vi "rqcAlice Pulse Detector And DAC Clock (FPGA).vi"(0 "delay line signal":bool, 1 "reset":bool, 2 "period":u8=40, 7 "DAC clock positions":T1=[0, 0]) -> (4 "DAC clock":bool, 6 "pusle arrived":bool)   [LabVIEW 2018]
uses:
  Custom Controls/Main State Machine/rqcAlice DAC Clock Positions.ctl
  <vilib>/RQC/FPGA Basic Logic/Counters/Counter (U8).vi
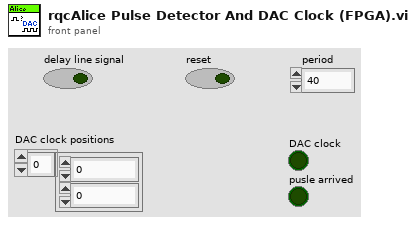
[diagram p1: front panel]
types:
  T1 = typedef "rqcAlice DAC Clock Positions.ctl" = u8[]
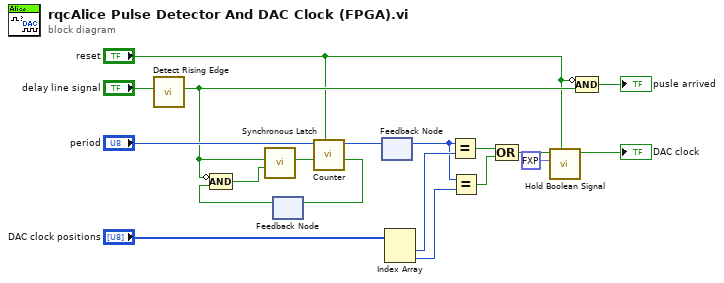
[diagram p0: block diagram]
diagram:
  n1 = call <vilib>:"Detect Rising Edge.vi"("signal"="delay line signal") -> ("edge detected"=w3:bool)  [unwired: 10 in]
  n2 = feedback #1() -> (w14:bool)  [unwired: 1 in]
  n3 = Compound Arithmetic op=AND(invert w3, w14) -> (w15:bool)
  n4 = call <vilib>:"Synchronous Latch.vi"("clear"=w15, "set"=w3) -> ("out"=w17:bool)  [unwired: 9 in]
  n5 = call-poly <vilib>:"Counter.vi"("reset"="reset", "increment"=w17, "bound"="period") -> ("done"=w16:bool, "count out"=w13:u8)  [unwired: 7 in]
  n6 = feedback-in #1(w16) -> ()
  n7 = feedback-in #2(w13) -> ()
  n8 = feedback #2() -> (w4:u8)  [unwired: 1 in]
  n9 = Index Array(array="DAC clock positions") -> (element #1=w12:u8, element #2=w11:u8)  [unwired: 2 in]
  n10 = Equal?(x=w4, y=w12) -> (x = y?=w10:bool)
  n11 = Equal?(x=w4, y=w11) -> (x = y?=w9:bool)
  n12 = Compound Arithmetic op=OR(w10, w9) -> (w8:bool)
  n13 = call <vilib>:"Hold Boolean Signal.vi"("reset"="reset", "width"=fxp<+,3,3> 5.0, "input signal"=w8) -> ("output signal"=→"DAC clock":bool)  [unwired: 8 in]
  n14 = Compound Arithmetic op=AND(invert "reset", w3) -> (→"pusle arrived":bool)
